vi "Haralick Features.vi"() -> ()   [LabVIEW 2016]
uses:
  <vilib>/vision/NI_Vision_Development_Module.lvlib
panel:
  out "IMG":T1(plugin-control)
  out "Feature Map":picture
  in  "Co-occurrence Options":T2={"  Level"=256, "Displacement Vector"={"xDelta"=1, "yDelta"=1}} {"Displacement Vector"."yDelta" min=1 step=1; "Displacement Vector"."xDelta" min=1 step=1}
  in  "Wavelet Options":T3={"Type"=14, "Wavelet Bands To Use"=[2], "Min. Energy Level"=100.0} {"Min. Energy Level" min=0 max=100; "Wavelet Bands To Use" items=["Low Low", "Low High", "High Low", "High High", "Low Low Low", "Low Low High", "Low High Low", "Low High High"]; "Type" items=["db02"=0, "db03"=1, "db04"=2, "db05"=3, "db06"=4, "db07"=5, "db08"=6, "db09"=7, "db10"=8, "db11"=9, "db12"=10, "db13"=11, "db14"=12, "Haar"=13, "bior1_3"=14, "bior1_5"=15, "bior2_2"=16, "bior2_4"=17, "bior2_6"=18, "bior2_8"=19, "bior3_1"=20, "bior3_3"=21, "bior3_5"=22, "bior3_7"=23, "bior3_9"=24, "bior4_4 (FBI)"=25, "bior5_5"=38, "bior6_8"=39, "coif1"=26, "coif2"=27, "coif3"=28, "coif4"=29, "coif5"=30, "sym2"=31, "sym3"=32, "sym4"=33, "sym5"=34, "sym6"=35, "sym7"=36, "sym8"=37]}
  in  "Window Options":T4={"SizeX"=32, "SizeY"=32, "Step Size"=0} {"Step Size" min=0 step=1; "SizeY" min=3 step=1; "SizeX" min=3 step=1}
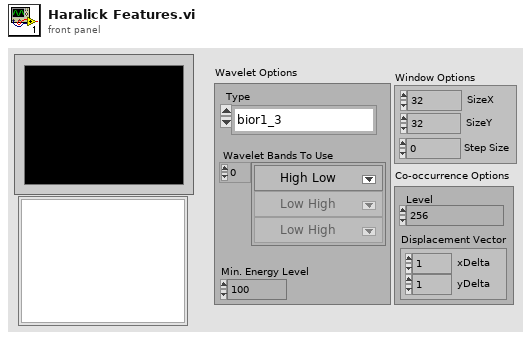
[diagram p1: front panel]
types:
  T1 = typedef "IMAQ Image.ctl" = refnum<image>
  T2 = cluster{"  Level":i32, "Displacement Vector":cluster{"xDelta":i32, "yDelta":i32}}
  T3 = cluster{"Type":i32, "Wavelet Bands To Use":i32[], "Min. Energy Level":sgl}
  T4 = cluster{"SizeX":i32, "SizeY":i32, "Step Size":i32}
  T5 = typedef "imagedata.ctl" = cluster{"image type":i32, "image depth":i32, "image":u8[], "mask":u8[], "colors":u32[], "Rectangle":cluster{"left":i16, "top":i16, "right":i16, "bottom":i16}}
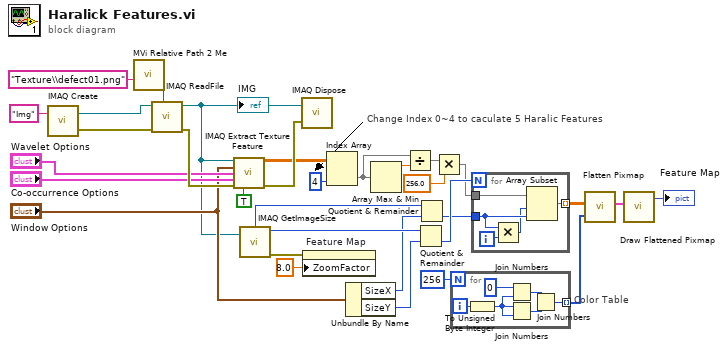
[diagram p0: block diagram]
diagram:
  # "Change Index 0~4 to caculate 5 Haralic Features"
  n1 = call "IMAQ Create"("Image Name"="Img") -> ("Src"=w29:T1, "error out"=w32:errorcluster)  [unwired: 4 in]
  n2 = call "MVi Relative Path 2 Me.vi"("Relative Path"="Texture\\defect01.png" ("name or relative path")) -> ("Appended Dir"=w1:path)  [unwired: 5 in, 1 out]
  n3 = call "IMAQ ReadFile"("File Path"=w1, "error in (no error)"=w32, "Image"=w29) -> ("error out"=w31:errorcluster, "Image Out"=w9:T1)  [unwired: 4 in, 3 out]
  "IMG" <- w9
  n4 = call "IMAQ Extract Texture Feature"("Image"=w9, "Window Options"="Window Options", "Wavelet Options"="Wavelet Options", "Co-occurrence Options"="Co-occurrence Options", "error in (no error)"=w31, "Use Window?"=TRUE) -> ("Texture Feature"=w23:dbl[][], "error out"=w30:errorcluster)  [unwired: 7 in, 1 out]
  n5 = call "IMAQ GetImageSize"("Image"=w9) -> ("Y Resolution"=w21:i32, "X Resolution"=w19:i32, "error out"=w16:errorcluster)  [unwired: 3 in]
  n6 = call "IMAQ Dispose"("Image"=w9, "error in (no error)"=w30) -> ()  [unwired: 4 in, 1 out]
  n7 = property on="Feature Map" class="Pict"(error in=w16, "ZoomFactor"=sgl 8.0 ("Zoom Factor")) -> ()  [unwired: 1 in, 2 out]
  n8 = Index Array(array=w23, index (col)=4 ("disabled index (col)")) -> (element=w5:dbl[])  [unwired: 1 in]
  n9 = Unbundle By Name("Window Options") -> ("SizeX"=w11:i32, "SizeY"=w10:i32)
  n10 = Array Max & Min(array=w5) -> (max value=w6:dbl)  [unwired: 3 out]
  n11 = Divide(x=w5, y=w6) -> (x/y=w7:dbl[])
  n12 = Quotient & Remainder(x=w21, y=w10) -> (floor(x/y)=w20:i32)  [unwired: 1 out]
  n13 = Quotient & Remainder(x=w19, y=w11) -> (floor(x/y)=w18:i32)  [unwired: 1 out]
  n14 = Multiply(x=w7, y=256.0) -> (x*y=w4:dbl[])
  n15 = for "Color Table" {
    N: 256 -> [_]
    tunnel: [w33] -> w15 mode=indexing
    i -> [w38]
    n16 = To Unsigned Byte Integer(number=w38) -> (unsigned 8bit integer=w37:u8)
    n17 = Join Numbers(hi=u8 0, lo=w37) -> ((hi.lo)=w35:u16)
    n18 = Join Numbers(hi=w37, lo=w37) -> ((hi.lo)=w34:u16)
    n19 = Join Numbers(hi=w35, lo=w34) -> ((hi.lo)=w33:u32)
  }
  n20 = for {
    N: w20 -> [_]
    tunnel: w4 -> [w43]
    tunnel: w18 -> [w41]
    tunnel: [w39] -> w3 mode=indexing
    i -> [w42]
    n21 = Multiply(x=w41, y=w42) -> (x*y=w40:i32)
    n22 = Array Subset(array=w43, index=w40, length=w41) -> (w39:dbl[])
  }
  n23 = call <vilib>:"Flatten Pixmap.vi"("colors"=w15, "8-bit pixmap"=w3) -> ("image data"=w14:T5)  [unwired: 9 in]
  n24 = call <vilib>:"Draw Flattened Pixmap.vi"("image data"=w14) -> ("new picture"=→"Feature Map":picture)  [unwired: 8 in]
